vi "Set Cell Data[i].vi"(8 "error in (no error)":errorcluster, 10 "Cell Data[i]":refnum<class "PAS Cell Data.lvclass">, 11 "PAS in":refnum<class "PAS.lvclass">) -> (0 "error out":errorcluster, 3 "PAS out":refnum<class "PAS.lvclass">)   [LabVIEW 2014, in "PAS.lvclass"]
uses:
  PAS.lvclass
  Data/Cell/PAS Cell Data.lvclass
  PAS.lvclass/PAS.ctl
  Data/Main/PAS Data.lvclass
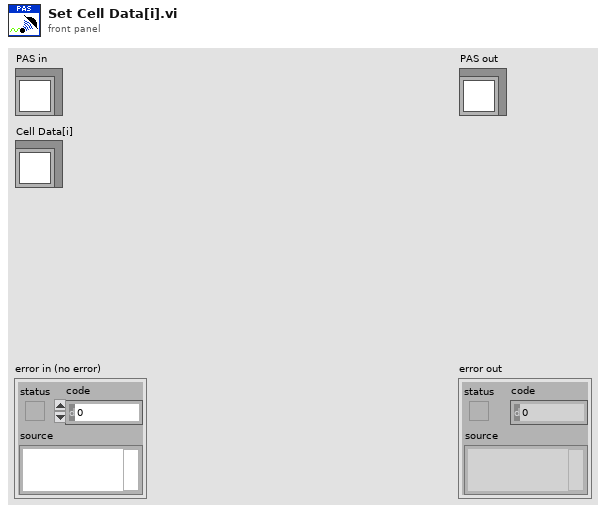
[diagram p1: front panel]
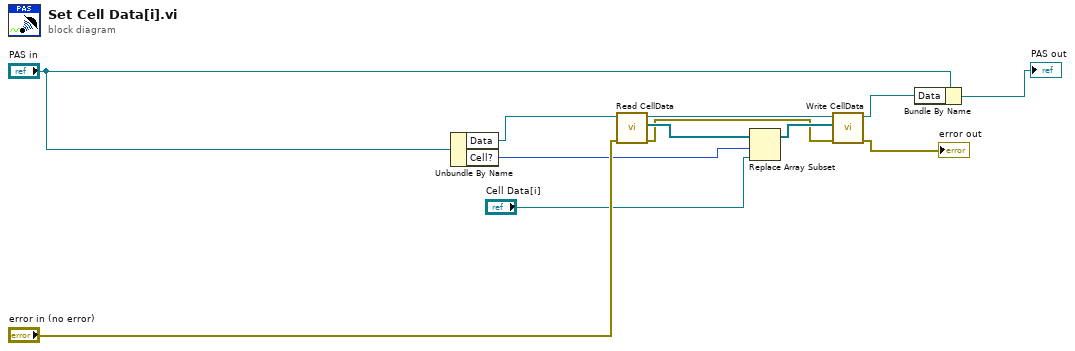
[diagram p0: block diagram]
diagram:
  n1 = Unbundle By Name("PAS in") -> ("Data"=w1:refnum<class "PAS Data.lvclass">, "Cell?"=w9:i32)
  n2 = call "Read CellData.vi"("error in"="error in (no error)", "PAS Data in"=w1) -> ("error out"=w5:errorcluster, "CellData"=w10:refnum<class "PAS Cell Data.lvclass">[], "PAS Data out"=w7:refnum<class "PAS Data.lvclass">)  [unwired: 7 in]
  n3 = Replace Array Subset(array=w10, new element="Cell Data[i]", index=w9) -> (w6:refnum<class "PAS Cell Data.lvclass">[])
  n4 = call "Write CellData.vi"("error in"=w5, "CellData"=w6, "PAS Data in"=w7) -> ("error out"=→"error out":errorcluster, "PAS Data out"=w3:refnum<class "PAS Data.lvclass">)  [unwired: 7 in]
  n5 = Bundle By Name(cluster="PAS in", "Data"=w3) -> (→"PAS out":refnum<class "PAS.lvclass">)
